vi "distributeVerticalCenters.vi"(6 "useControlBodyOnly":bool, 7 "horizontalAlignment":T1, 8 "error in (no error)":errorcluster, 11 "refs":refnum<vi>[](array[refnum])) -> (0 "error out":errorcluster, 3 "refs(dup)":refnum<vi>[](array[refnum]))   [LabVIEW 2023]
doc: "Arranges the input controls vertically, making their centers equidistant. The topmost and bottommost centers are kept fixed, while the other centers are distributed in between.\nThe horizontal position is processed according to the input 'horizontalArrangement'."
uses:
  Ctrls/alignment.ctl
  Misc/processUseControlBodyOnlyFlag_start.vi
  Misc/processUseControlBodyOnlyFlag_end.vi
  Misc/hideCaption&Label.vi
  Misc/setCaption&LabelVisibility.vi
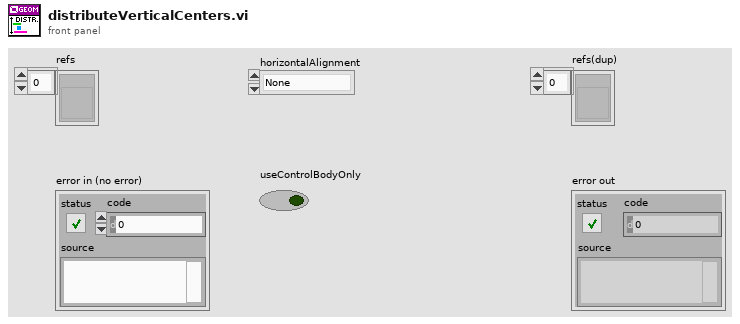
[diagram p1: front panel]
types:
  T1 = typedef "alignment.ctl" = enum16{"None", "AlignTop", "AlignBottom", "AlignHorizontalCenters", "AlignLeft", "AlignRight", "AlignVerticalCenters"}
  T2 = cluster{"left":i32, "top":i32, "right":i32, "bottom":i32}
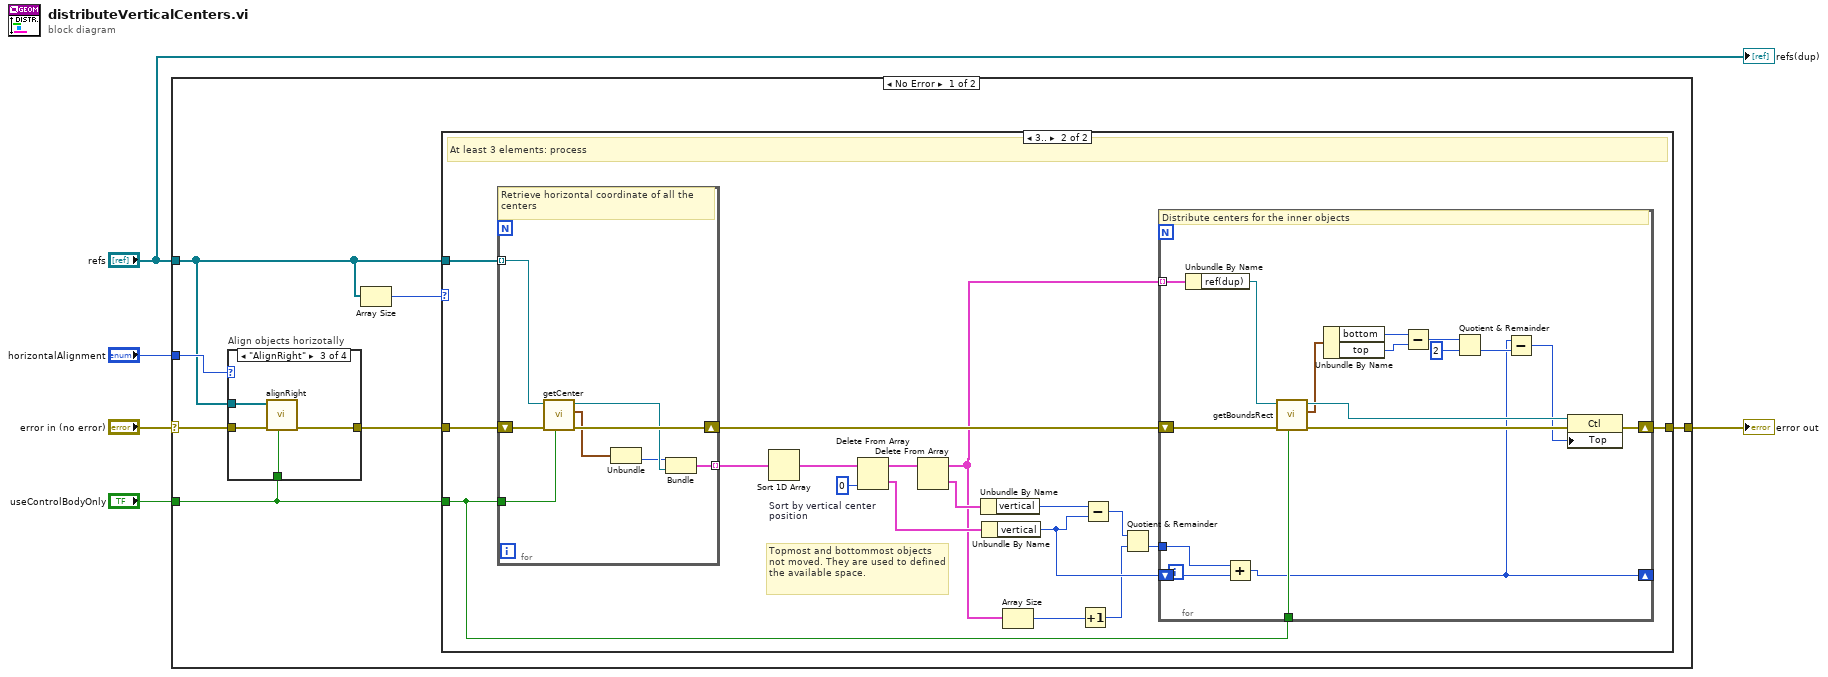
[diagram p0: block diagram]
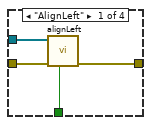
[diagram p3: hidden frame]
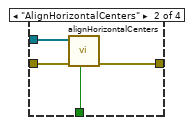
[diagram p4: hidden frame]
diagram:
  n1 = case shown="No Error" "error in (no error)" {
    selector: "error in (no error)" -> [w11 w70]
    tunnel: [w12 w70] -> w2
    tunnel: "refs" -> [w7 _]
    tunnel: "useControlBodyOnly" -> [w9 _]
    tunnel: "horizontalAlignment" -> [w8 _]
    frame No Error {
      n2 = case "Align objects horizotally" shown="\"AlignRight\"" w8 {
        tunnel: w11 -> [w60 w64 w68 w69]
        tunnel: [w59 w63 w67 w69] -> w10
        tunnel: w9 -> [w58 w62 w66 _]
        tunnel: w7 -> [w57 w61 w65 _]
        frame "AlignLeft" {
          n3 = call "alignLeft.vi"("useControlBodyOnly"=w58, "error in (no error)"=w60, "refs"=w57) -> ("error out"=w59:errorcluster)  [unwired: 7 in, 1 out]
        }
        frame "AlignHorizontalCenters" {
          n4 = call "alignHorizontalCenters.vi"("useControlBodyOnly"=w62, "error in (no error)"=w64, "refs"=w61) -> ("error out"=w63:errorcluster)  [unwired: 7 in, 1 out]
        }
        frame "AlignRight" {
          n5 = call "alignRight.vi"("useControlBodyOnly"=w66, "error in (no error)"=w68, "refs"=w65) -> ("error out"=w67:errorcluster)  [unwired: 7 in, 1 out]
        }
        frame "None", Default {
        }
      }
      n6 = Array Size(array=w7) -> (size(s)=w6:i32)
      n7 = case shown="3.." w6 {
        tunnel: [w13 w21] -> w12
        tunnel: w10 -> [w13 w31]
        tunnel: w9 -> [_ w20]
        tunnel: w7 -> [_ w30]
        frame ..2 {
          # "Not enough elements: do nothing"
        }
        frame 3.. {
          # "Topmost and bottommost objects not moved. They are used to defined the available space."
          # "At least 3 elements: process"
          n8 = for {
            shift-right: [w55] -> w22
            shift-left: w31 -> [w56]
            tunnel: w30 -> [w53] mode=indexing
            tunnel: w20 -> [w54]
            tunnel: [w50] -> w29 mode=indexing
            # "Retrieve horizontal coordinate of all the centers"
            n9 = call "getCenter.vi"("useControlBodyOnly"=w54, "error in (no error)"=w56, "ref"=w53) -> ("error out"=w55:errorcluster, "center"=w52:cluster{"horizontal":i32, "vertical":i32}, "ref(dup)"=w51:refnum<vi>)  [unwired: 6 in]
            n10 = Unbundle(w52) -> ("vertical"=w49:i32)  [unwired: 1 out]
            n11 = Bundle("vertical"=w49, "ref(dup)"=w51) -> (w50:cluster{"vertical":i32, "ref(dup)":refnum<vi>})  [unwired: 1 in]
          }
          n12 = Sort 1D Array "Sort by vertical center position"(array=w29) -> (sorted array=w17:cluster{"vertical":i32, "ref(dup)":refnum<vi>}[])
          n13 = Delete From Array(array=w17, index=0) -> (deleted portion=w25:cluster{"vertical":i32, "ref(dup)":refnum<vi>}, array with subset deleted=w27:cluster{"vertical":i32, "ref(dup)":refnum<vi>}[])  [unwired: 1 in]
          n14 = Delete From Array(array=w27) -> (deleted portion=w26:cluster{"vertical":i32, "ref(dup)":refnum<vi>}, array with subset deleted=w16:cluster{"vertical":i32, "ref(dup)":refnum<vi>}[])  [unwired: 2 in]
          n15 = Unbundle By Name(w26) -> ("vertical"=w24:i32)
          n16 = Unbundle By Name(w25) -> ("vertical"=w18:i32)
          n17 = Array Size(array=w16) -> (size(s)=w15:i32)
          n18 = Increment(x=w15) -> (x+1=w14:i32)
          n19 = Subtract(x=w24, y=w18) -> (x-y=w23:i32)
          n20 = Quotient & Remainder(x=w23, y=w14) -> (floor(x/y)=w19:i32)  [unwired: 1 out]
          n21 = for {
            shift-right: [w37] -> w21
            shift-left: w22 -> [w38]
            tunnel: w19 -> [w33]
            tunnel: w16 -> [w48] mode=indexing
            tunnel: w20 -> [w35]
            shift-right: [w32] -> _
            shift-left: w18 -> [w34]
            # "Distribute centers for the inner objects"
            n22 = Unbundle By Name(w48) -> ("ref(dup)"=w36:refnum<vi>)
            n23 = Add(x=w33, y=w34) -> (x+y=w32:i32)
            n24 = call "getBoundsRect.vi"("useControlBodyOnly"=w35, "error in (no error)"=w38, "ref"=w36) -> ("error out"=w43:errorcluster, "rect"=w41:T2, "ref(dup)"=w42:refnum<vi>)  [unwired: 6 in]
            n25 = Unbundle By Name(w41) -> ("bottom"=w47:i32, "top"=w46:i32)
            n26 = Subtract(x=w47, y=w46) -> (x-y=w44:i32)
            n27 = Quotient & Remainder(x=w44, y=2) -> (floor(x/y)=w45:i32)  [unwired: 1 out]
            n28 = Subtract(x=w32, y=w45) -> (x-y=w39:i32)
            n29 = property class="Ctl"(reference=w42, error in=w43, "Top"=w39) -> (error out=w37:errorcluster)  [unwired: 1 out]
          }
        }
      }
    }
    frame Error {
    }
  }
  "error out" <- w2
  "refs(dup)" <- "refs"
